vi "To String.vi"(8 "error in (no error)":errorcluster, 11 "Enum Array in":refnum<class "Enum Array.lvclass">) -> (0 "error out":errorcluster, 2 "String":string)   [LabVIEW 2020, in "Data.lvlib" / "Enum Array.lvclass"]
doc: "Convert 'Generic Data in' to a string."
uses:
  Enum Array.lvclass
  Enum Array.lvclass/Enum Array.ctl
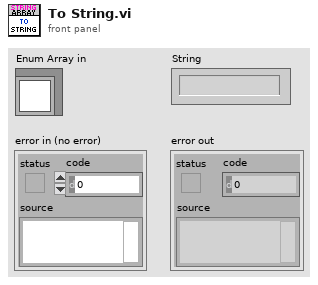
[diagram p1: front panel]
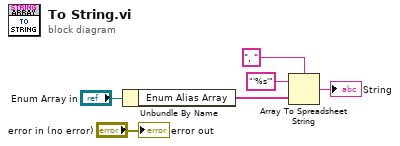
[diagram p0: block diagram]
diagram:
  n1 = Unbundle By Name("Enum Array in") -> ("Enum Alias Array"=w1:string[])
  n2 = Array To Spreadsheet String(delimiter (Tab)=", ", array=w1, 3:"'%s'" ("format string")) -> (spreadsheet string=→"String":string)
  "error out" <- "error in (no error)"
